vi "Lifter.vi"(0 "Button 6 up":bool, 1 "Button 7 down":bool, 2 "Button 11 up":bool, 3 "Button 10 down":bool, 4 "top left":bool, 5 "top right":bool, 6 "bottom left":bool, 7 "bottom right":bool) -> ()   [LabVIEW 2012]
uses:
  <vilib>/Rock Robotics/WPI/Relay/WPI_RelayValue.ctl
panel:
  in  "Lifter 2 On?":bool
  in  "Lifter 1 On?":bool
  out "Launcher On?":bool
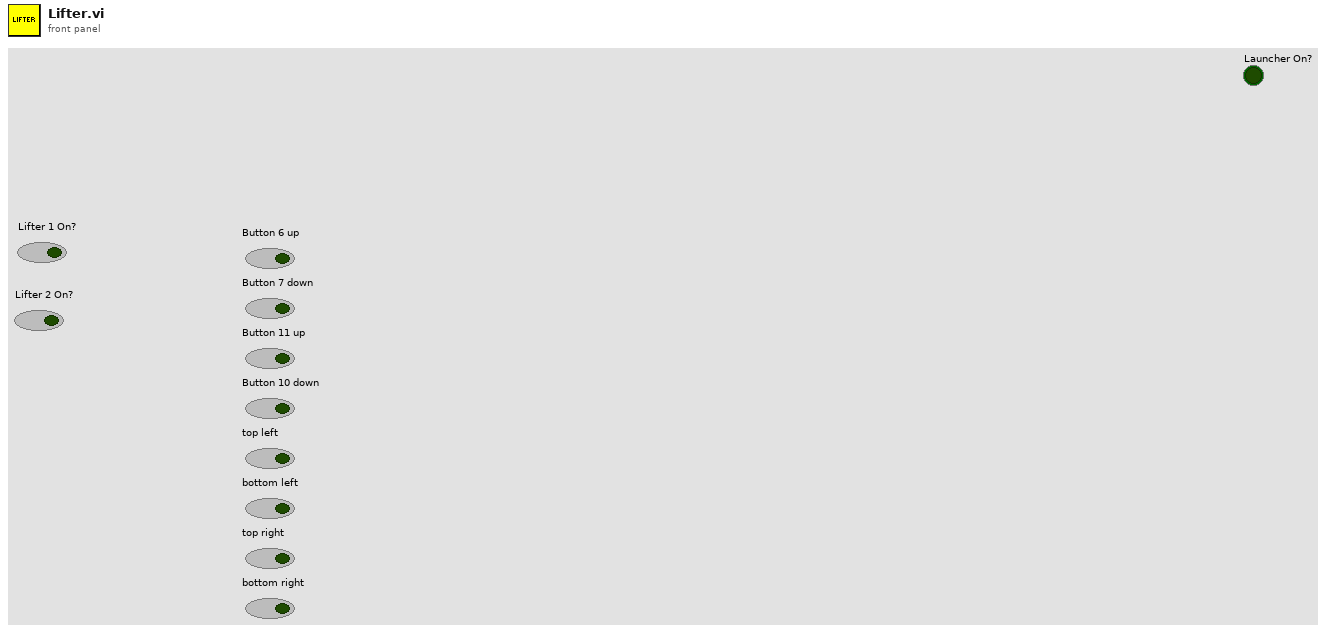
[diagram p1: front panel]
types:
  T1 = typedef "WPI_RelayValue.ctl" = enum16{"Off", "On", "Forward", "Reverse"}
  T2 = typedef "WPI_RelayDevRef.ctl" = cluster{"DevStatus":errorcluster, "Relay Channel":T3, "Digital Module":T4, "Relay Direction":T5}
  T3 = typedef "FPGA_DIORelayChannel.ctl" = enum8{"Relay 1", "Relay 2", "Relay 3", "Relay 4", "Relay 5", "Relay 6", "Relay 7", "Relay 8", "Invalid"}
  T4 = typedef "FPGA_TypedefDigitalModule.ctl" = enum16{"Digital Module 1", "Digital Module 2"}
  T5 = typedef "WPI_RelayDirection.ctl" = enum16{"Both directions", "Forward only", "Reverse only"}
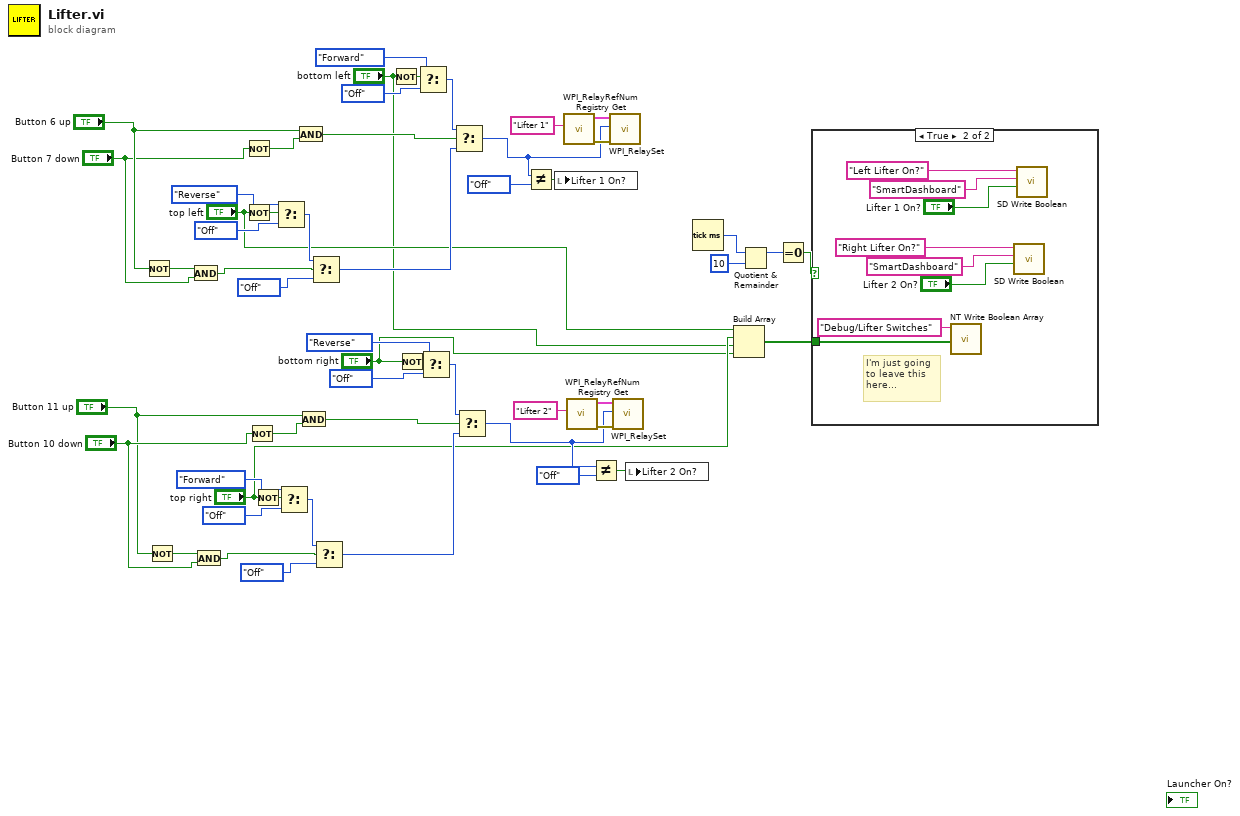
[diagram p0: block diagram]
diagram:
  n1 = Not(x="Button 6 up") -> (.not. x?=w48:bool)
  n2 = Not(x="Button 11 up") -> (.not. x?=w26:bool)
  n3 = And(x=w48, y="Button 7 down") -> (x .and. y?=w7:bool)
  n4 = And(x=w26, y="Button 10 down") -> (x .and. y?=w28:bool)
  n5 = Not(x="Button 7 down") -> (.not. x?=w50:bool)
  n6 = Not(x="top left") -> (.not. x?=w19:bool)
  n7 = Not(x="Button 10 down") -> (.not. x?=w24:bool)
  n8 = Not(x="top right") -> (.not. x?=w18:bool)
  n9 = Select(t=WPI_RelayValue."Reverse" ("RelayValue"), s=w19, f=WPI_RelayValue."Off") -> (s? t:f=w42:T1)
  n10 = Select(t=WPI_RelayValue."Forward" ("RelayValue"), s=w18, f=WPI_RelayValue."Off") -> (s? t:f=w33:T1)
  n11 = And(x="Button 6 up", y=w50) -> (x .and. y?=w49:bool)
  n12 = And(x="Button 11 up", y=w24) -> (x .and. y?=w25:bool)
  n13 = Select(t=w42, s=w7, f=WPI_RelayValue."Off" ("RelayValue")) -> (s? t:f=w44:T1)
  n14 = Select(t=w33, s=w28, f=WPI_RelayValue."Off" ("RelayValue")) -> (s? t:f=w31:T1)
  n15 = Not(x="bottom left") -> (.not. x?=w20:bool)
  n16 = Not(x="bottom right") -> (.not. x?=w17:bool)
  n17 = Select(t=WPI_RelayValue."Forward" ("RelayValue"), s=w20, f=WPI_RelayValue."Off") -> (s? t:f=w39:T1)
  n18 = Select(t=WPI_RelayValue."Reverse" ("RelayValue"), s=w17, f=WPI_RelayValue."Off") -> (s? t:f=w36:T1)
  n19 = Select(t=w39, s=w49, f=w44) -> (s? t:f=w10:T1)
  n20 = Select(t=w36, s=w25, f=w31) -> (s? t:f=w13:T1)
  n21 = Not Equal?(x=w10, y=WPI_RelayValue."Off") -> (x != y?=w9:bool)
  n22 = local write "Lifter 1 On?"(w9) -> ()
  n23 = call <vilib>:"WPI_RelayRefNum Registry Get.vi"("refnum name"="Lifter 1") -> ("error out"=w53:errorcluster, "RelayDevRef"=w52:T2)  [unwired: 9 in]
  n24 = call <vilib>:"WPI_RelayRefNum Registry Get.vi"("refnum name"="Lifter 2") -> ("error out"=w21:errorcluster, "RelayDevRef"=w22:T2)  [unwired: 9 in]
  n25 = Not Equal?(x=w13, y=WPI_RelayValue."Off") -> (x != y?=w11:bool)
  n26 = call <vilib>:"WPI_RelaySet.vi"("error in (no error)"=w53, "RelayValue"=w10, "RelayDevRef"=w52) -> ()  [unwired: 7 in, 2 out]
  n27 = call <vilib>:"WPI_RelaySet.vi"("error in (no error)"=w21, "RelayValue"=w13, "RelayDevRef"=w22) -> ()  [unwired: 7 in, 2 out]
  n28 = local write "Lifter 2 On?"(w11) -> ()
  n29 = Tick Count (ms)() -> (millisecond timer value=w16:u32)
  n30 = Build Array("top left", "top right", "bottom left", "bottom right") -> (w1:bool[])
  n31 = Quotient & Remainder(x=w16, y=u32 10) -> (x-y*floor(x/y)=w15:u32)  [unwired: 1 out]
  n32 = Equal To 0?(x=w15) -> (x = 0?=w14:bool)
  n33 = case shown="True" w14 {
    tunnel: w1 -> [_ w55]
    frame False {
    }
    frame True {
      # "I'm just going\nto leave this\nhere..."
      n34 = call <vilib>:"NT Write Boolean Array.vi"("Boolean Array"=w55, "Name"="Debug/Lifter Switches") -> ()  [unwired: 9 in, 1 out]
      n35 = call <vilib>:"SD Write Boolean.vi"("Boolean"="Lifter 2 On?", "Table Prefix"="SmartDashboard", "Name"="Right Lifter On?") -> ()  [unwired: 7 in, 2 out]
      n36 = call <vilib>:"SD Write Boolean.vi"("Boolean"="Lifter 1 On?", "Table Prefix"="SmartDashboard", "Name"="Left Lifter On?") -> ()  [unwired: 7 in, 2 out]
    }
  }
